vi "DjtgGetTdoBits.vi"(4 "TMS State":u8, 6 "TDI State":u8, 7 "Overlap?":bool, 8 "Error In":errorcluster, 9 "Num Pit Pairs":u32, 10 "Data Buffer Size (bytes)":i32=4, 11 "Device Number":u32) -> (0 "Error Out":errorcluster, 2 "Data":u8[](array[numeric]), 3 "Device Number":u32)   [LabVIEW 2011, in "LVH-Adept.lvlib" / "DJTG.lvlib"]
doc: "When the DJTG port is configured for JScan0, JScan1, JScan2, or JScan3 the fTdi and fTms parameters specify the state at which the TDIC and TMSC pins are held for the duration of the data transfer. When the DJTG port is configured for any other scan format the fTdi and fTms parameters specify whether a ‘1’ or a ‘0’ is output on the TMSC pin for each TDI and TMS bit in the scan packet. If the scan format that the port is currently configured for doesn’t contain any TDI bits then the fTdi parameter is ignored. Similarly, if the scan format doesn’t contain any TMS bits then the fTms parameter is ignored."
uses:
  DJTG.lvlib
  Private/Type Defs/Error.ctl
  <vilib>/LabVIEW Hacker/Adept/Private/Resources/djtg.dll
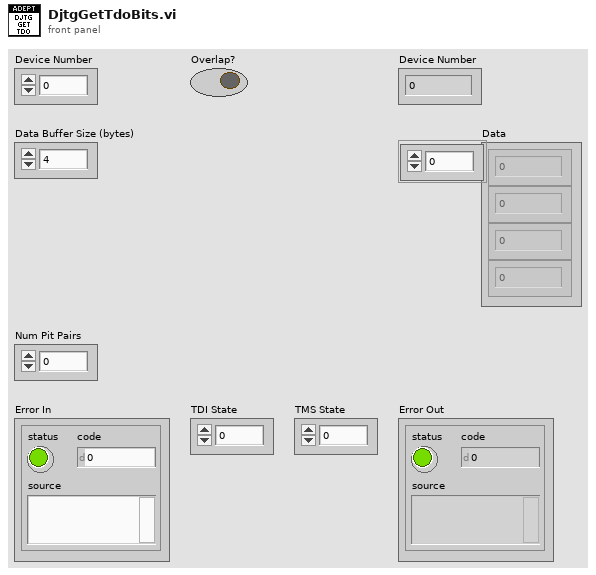
[diagram p1: front panel]
types:
  T1 = typedef "LVH-Adept.lvlib/DJTG.lvlib/Error.ctl" = enum16{"Unknown", "Enable", "PutTmsTdiBits", "GetTdoBits", "Disable", "Close", "Set Aux Reset", "Port Properties", "Get Speed", "Set Speed", "Get Port Count", "Get Batch Properties", "Enable Port", "Set Tmd Tdi Tck", "Get Tms Tdi Tdo Tck", "Put Tdi Bits", "Put Tms Bits", "Clock Tck", "Wait", "Batch", "Flash FPGA"}
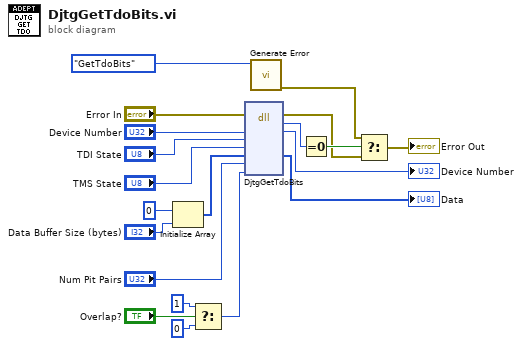
[diagram p0: block diagram]
diagram:
  n1 = Initialize Array(u8 0, "Data Buffer Size (bytes)") -> (w1:u8[])
  n2 = Select(t=u8 1, s="Overlap?", f=u8 0) -> (s? t:f=w7:u8)
  n3 = dll-call lib="C:/Program Files (x86)/National Instruments/LabVIEW 2011/vi.lib/LabVIEW Hacker/Adept/Private/Resources/djtg.dll" fn="DjtgGetTdoBits"(error in="Error In", "HIF"="Device Number", "fTdi"="TDI State", "fTms"="TMS State", "rgbRcv"=w1, "cbits"="Num Pit Pairs", "fOverlap"=w7) -> (error out=w16:errorcluster, "Success"=w18:u32, "HIF"=→"Device Number":u32, "rgbRcv"=→"Data":u8[])  [unwired: 6 in, 1 out]
  n4 = call "Generate Error.vi"("DJTG Error"=Error."GetTdoBits") -> ("Error Out"=w17:errorcluster)  [unwired: 10 in]
  n5 = Equal To 0?(x=w18) -> (x = 0?=w19:bool)
  n6 = Select(t=w17, s=w19, f=w16) -> (s? t:f=→"Error Out":errorcluster)
